vi "Build Valley.vi"(1 "Puzzle Input":string) -> (0 "Valley":T1[][](array[typedef]))   [LabVIEW 2020, in "AoC 2022.lvlib"]
uses:
  AoC 2022.lvlib
  Valley Item.ctl
  Valley Point.ctl
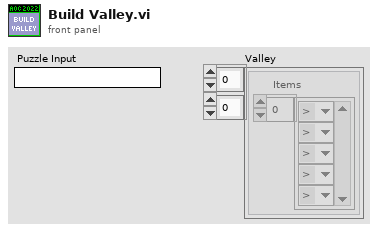
[diagram p1: front panel]
types:
  T1 = typedef "AoC 2022.lvlib/Valley Point.ctl" = cluster{"Items":T2[]}
  T2 = typedef "AoC 2022.lvlib/Valley Item.ctl" = enum16{"#", ".", ">", "<", "^", "v", "E"}
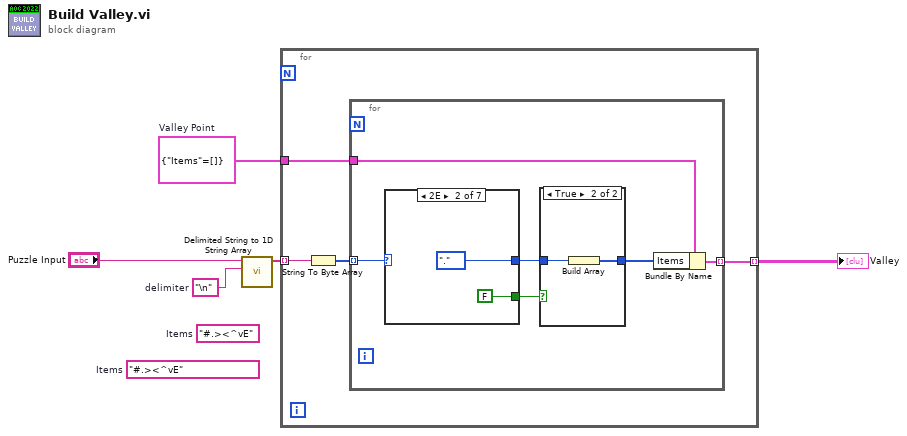
[diagram p0: block diagram]
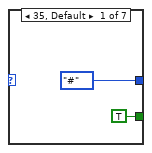
[diagram p3: hidden frame]
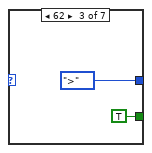
[diagram p4: hidden frame]
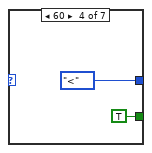
[diagram p5: hidden frame]
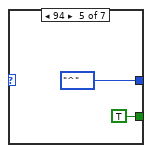
[diagram p6: hidden frame]
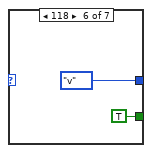
[diagram p7: hidden frame]
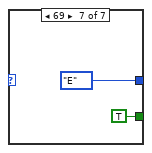
[diagram p8: hidden frame]
diagram:
  (unwired) "#.><^vE"  # Items
  (unwired) "#.><^vE"  # Items
  w4 = T1 {"Items"=[]}  # Valley Point
  w2 = "\n"  # delimiter
  n1 = call <vilib>:"Delimited String to 1D String Array.vi"("delimiter"=w2, "delimited string"="Puzzle Input") -> ("string array"=w3:string[])  [unwired: 9 in]
  n2 = for {
    tunnel: w3 -> [w9] mode=indexing
    tunnel: w4 -> [w7]
    tunnel: [w6] -> w5 mode=indexing
    n3 = String To Byte Array(string=w9) -> (unsigned byte array=w8:u8[])
    n4 = for {
      tunnel: w8 -> [w15] mode=indexing
      tunnel: w7 -> [w14]
      tunnel: [w11] -> w6 mode=indexing
      n5 = case shown="2E" w15 {
        tunnel: [Valley_Item."#" ("Blizzard") Valley_Item."." ("Blizzard") Valley_Item.">" ("Blizzard") Valley_Item."<" ("Blizzard") Valley_Item."^" ("Blizzard") Valley_Item."v" ("Blizzard") Valley_Item."E" ("Blizzard")] -> w12
        tunnel: [TRUE FALSE TRUE TRUE TRUE TRUE TRUE] -> w10
        frame 35, Default {
        }
        frame 46 {
        }
        frame 62 {
        }
        frame 60 {
        }
        frame 94 {
        }
        frame 118 {
        }
        frame 69 {
        }
      }
      n6 = case shown="True" w10 {
        tunnel: [_ w17] -> w13
        tunnel: w12 -> [_ w16]
        frame False {
        }
        frame True {
          n7 = Build Array(w16) -> (w17:T2[])
        }
      }
      n8 = Bundle By Name(cluster=w14, "Items"=w13) -> (w11:T1)
    }
  }
  "Valley" <- w5
